vi "Modbus.Connect.vi"(8 "error in (no error)":errorcluster, 11 "Config":T1={"address"="", "port (502)"=502, "connect timeout ms"=10000}) -> (0 "error out":errorcluster)   [LabVIEW 2019, in "Modbus.lvlib"]
uses:
  Modbus.lvlib
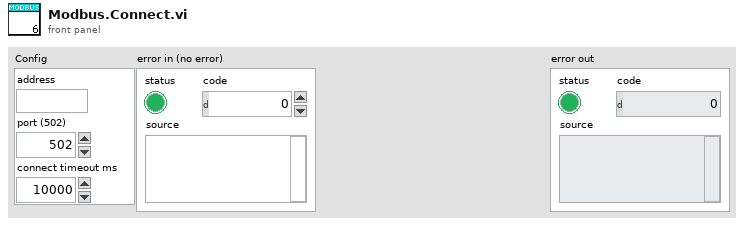
[diagram p1: front panel]
types:
  T1 = cluster{"address":string, "port (502)":u16, "connect timeout ms":i32}
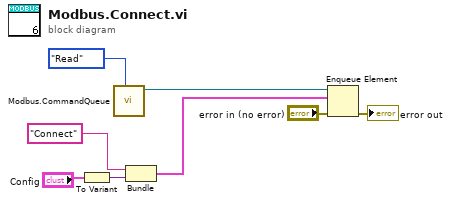
[diagram p0: block diagram]
diagram:
  n1 = To Variant(anything="Config") -> (Variant=w3:variant)
  n2 = call "Modbus.CommandQueue.vi"("OP"=enum16{"Read", "Write"}."Read") -> ("queue OUT"=w7:refnum<queue>)  [unwired: 10 in]
  n3 = Bundle("Connect", "Variant"=w3) -> (w4:cluster{string, "Variant":variant})  [unwired: 1 in]
  n4 = Enqueue Element(queue=w7, element=w4, error in (no error)="error in (no error)") -> (error out=→"error out":errorcluster)  [unwired: 1 in, 2 out]
